vi "GetCetoniPump.vi"(0 "object in":refnum<class "Application.lvclass">, 5 "error in (no error)":errorcluster) -> (14 "object out":refnum<class "Application.lvclass">, 15 "CetoniPump":refnum<class "CetoniPump.lvclass">, 19 "error out":errorcluster)   [LabVIEW 2021, in "Application.lvclass"]
uses:
  Application.lvclass
  Application.lvclass/Application.ctl
  CetoniPump_class/CetoniPump.lvclass
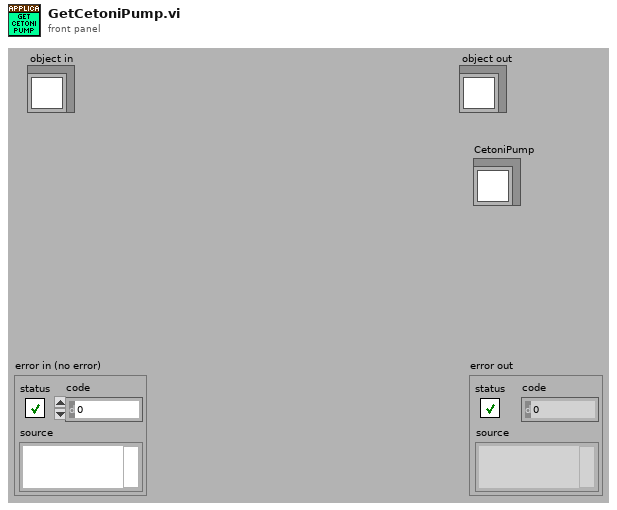
[diagram p1: front panel]
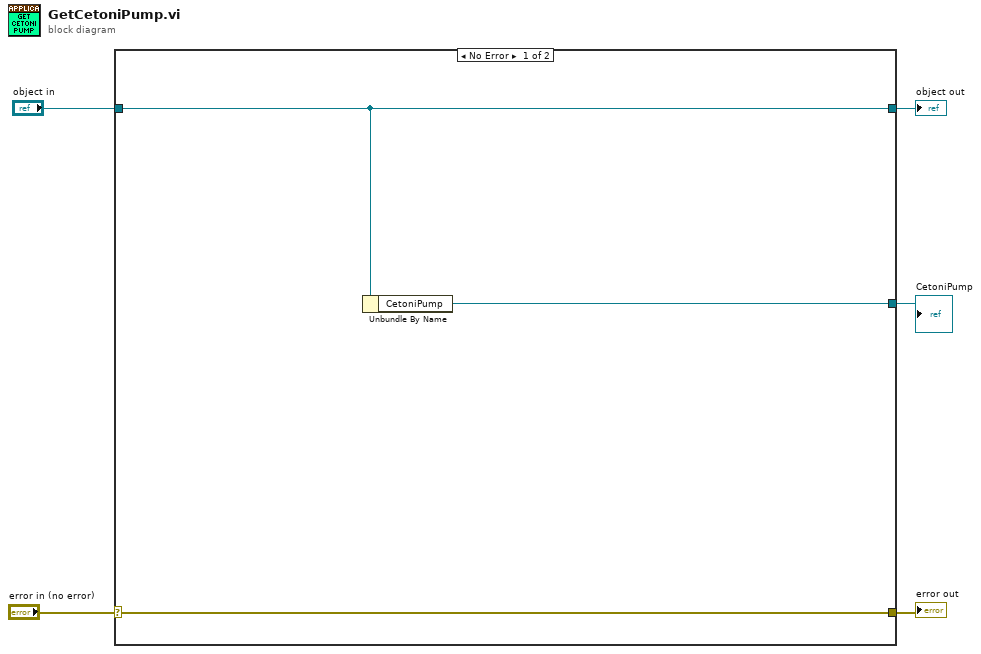
[diagram p0: block diagram]
diagram:
  n1 = case shown="No Error" "error in (no error)" {
    selector: "error in (no error)" -> [w7 w10]
    tunnel: [w7 w10] -> w4
    tunnel: [w6 w9] -> w2
    tunnel: "object in" -> [w6 w9]
    tunnel: [w8 _] -> w1
    frame No Error {
      n2 = Unbundle By Name(w6) -> ("CetoniPump"=w8:refnum<class "CetoniPump.lvclass">)
    }
    frame Error {
    }
  }
  "error out" <- w4
  "object out" <- w2
  "CetoniPump" <- w1
